vi "AndorTester.vi"() -> ()   [LabVIEW 2014]
uses:
  <userlib>/atmcd32d/Error Code Enum typedef.ctl
  <userlib>/atmcd32d/ReadMode_mode typedef.ctl
  <userlib>/atmcd32d/AcquisitionMode_mode typedef.ctl
panel:
  in  "set temp":i32
  out "status":T1
  out "temperature":i32
  out "Numeric":i32
  out "size(s)":i32
  out "Waveform Chart":i32[](graph)
  in  "stop":bool
  out "Current camera":i32
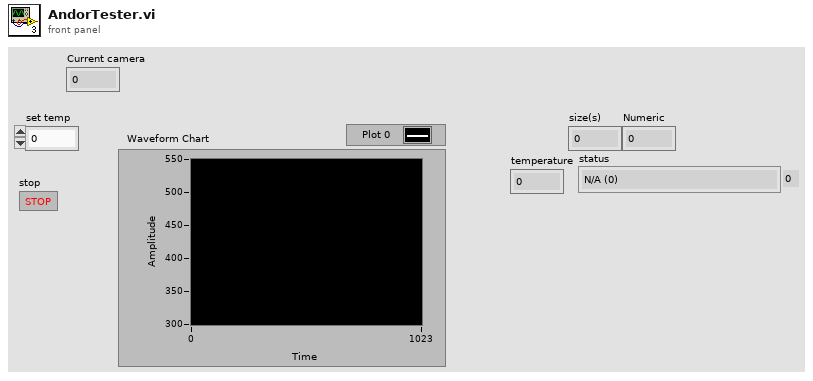
[diagram p1: front panel]
types:
  T1 = typedef "Error Code Enum typedef.ctl" = enum32{"N/A (0)", "DRV_ERROR_CODES", "DRV_SUCCESS", "DRV_VXDNOTINSTALLED", "DRV_ERROR_SCAN", "DRV_ERROR_CHECK_SUM", "DRV_ERROR_FILELOAD", "DRV_UNKNOWN_FUNC", "DRV_ERROR_VXD_INIT", "DRV_ERROR_ADDRESS", "DRV_ERROR_PAGELOCK", "DRV_ERROR_PAGEUNLOCK", "DRV_ERROR_BOARDTEST", "DRV_ERROR_ACK", "DRV_ERROR_UP_FIFO", "DRV_ERROR_PATTERN", "N/A (16)", "DRV_ACQUISITION_ERRORS", "DRV_ACQ_BUFFER", "DRV_ACQ_DOWNFIFO_FULL", "DRV_PROC_UNKONWN_INSTRUCTION", "DRV_ILLEGAL_OP_CODE", "DRV_KINETIC_TIME_NOT_MET", "DRV_ACCUM_TIME_NOT_MET", "DRV_NO_NEW_DATA", "N/A (25)", "DRV_SPOOLERROR", "N/A (27)", "N/A (28)", "N/A (29)", "N/A (30)", "N/A (31)", "N/A (32)", "DRV_TEMPERATURE_CODES", "DRV_TEMPERATURE_OFF", "DRV_TEMPERATURE_NOT_STABILIZED", "DRV_TEMPERATURE_STABILIZED", "DRV_TEMPERATURE_NOT_REACHED", "DRV_TEMPERATURE_OUT_RANGE", "DRV_TEMPERATURE_NOT_SUPPORTED", "DRV_TEMPERATURE_DRIFT", "N/A (41)", "N/A (42)", "N/A (43)", "N/A (44)", "N/A (45)", "N/A (46)", "N/A (47)", "N/A (48)", "DRV_GENERAL_ERRORS", "DRV_INVALID_AUX", "DRV_COF_NOTLOADED", "DRV_FPGAPROG", "DRV_FLEXERROR", "DRV_GPIBERROR", "N/A (55)", "N/A (56)", "N/A (57)", "N/A (58)", "N/A (59)", "N/A (60)", "N/A (61)", "N/A (62)", "N/A (63)", "DRV_DATATYPE", "DRV_DRIVER_ERRORS", "DRV_P1INVALID", "DRV_P2INVALID", "DRV_P3INVALID", "DRV_P4INVALID", "DRV_INIERROR", "DRV_COFERROR", "DRV_ACQUIRING", "DRV_IDLE", "DRV_TEMPCYCLE", "DRV_NOT_INITIALIZED", "DRV_P5INVALID", "DRV_P6INVALID", "DRV_INVALID_MODE", "DRV_INVALID_FILTER", "DRV_I2CERRORS", "DRV_I2CDEVNOTFOUND", "DRV_I2CTIMEOUT", "DRV_P7INVALID", "N/A (84)", "N/A (85)", "N/A (86)", "N/A (87)", "N/A (88)", "N/A (89)", "DRV_IOCERROR", "DRV_VRMVERSIONERROR"}
  T2 = typedef "AcquisitionMode_mode typedef.ctl" = enum16{"Reserved (0)", "Single Scan", "Accumulate", "Kinetics", "Fast Kinetics", "Run Till Abort", "Reserved (6)", "Reserved (7)", "Reserved (8)", "Time Delayed Integration"}
  T3 = typedef "ReadMode_mode typedef.ctl" = enum16{"Full Vertical Binning", "Multi-Track", "Random-Track", "Single-Track", "Image"}
  T4 = typedef "IMAQ Image.ctl" = refnum<image>
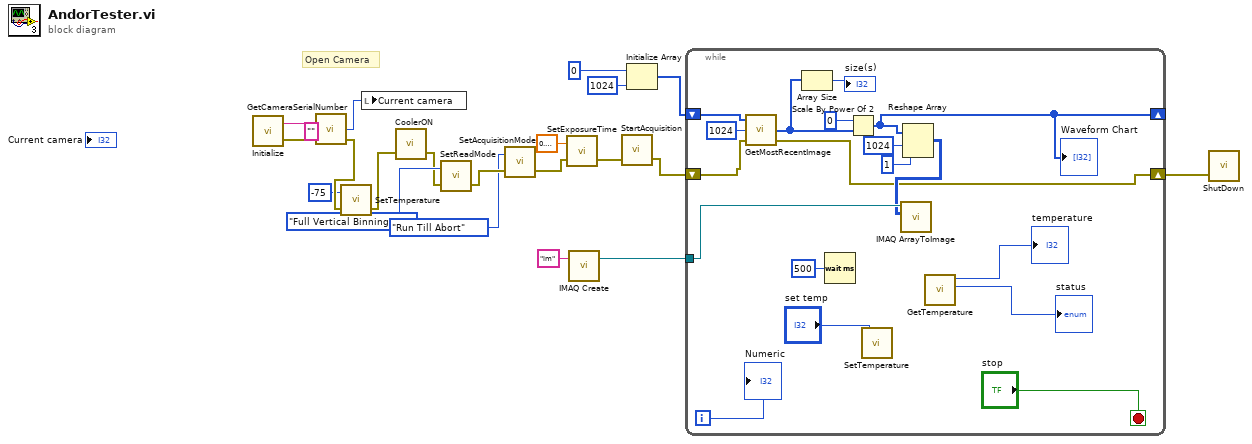
[diagram p0: block diagram]
diagram:
  # "Open Camera"
  n1 = call <userlib>:"Initialize.vi"("directory (\"\")"="" ("directory (\"\")")) -> ("error out"=w18:errorcluster)  [unwired: 1 in, 1 out]
  n2 = call <userlib>:"GetCameraSerialNumber.vi"("error in (no error)"=w18) -> ("error out"=w3:errorcluster, "number"=w19:i32)  [unwired: 2 in, 1 out]
  n3 = call <userlib>:"SetTemperature.vi"("error in (no error)"=w3, "temperature"=-75) -> ("error out"=w2:errorcluster)  [unwired: 1 out]
  n4 = local write "Current camera"(w19) -> ()
  n5 = call <userlib>:"CoolerON.vi"("error in (no error)"=w2) -> ("error out"=w4:errorcluster)  [unwired: 1 in, 1 out]
  n6 = call <userlib>:"SetReadMode.vi"("error in (no error)"=w4, "mode"=ReadMode_mode_typedef."Full Vertical Binning") -> ("error out"=w10:errorcluster)  [unwired: 1 out]
  n7 = call <userlib>:"SetAcquisitionMode.vi"("error in (no error)"=w10, "mode"=AcquisitionMode_mode_typedef."Run Till Abort") -> ("error out"=w7:errorcluster)  [unwired: 1 out]
  n8 = call <userlib>:"SetExposureTime.vi"("error in (no error)"=w7, "time"=sgl 0.3) -> ("error out"=w6:errorcluster)  [unwired: 1 out]
  n9 = call "IMAQ Create"("Image Name"="im") -> ("New Image"=w17:T4)  [unwired: 4 in, 1 out]
  n10 = call <userlib>:"StartAcquisition.vi"("error in (no error)"=w6) -> ("error out"=w5:errorcluster)  [unwired: 1 in, 1 out]
  n11 = Initialize Array(0, 1024 ("dimension size")) -> (w13:i32[])
  n12 = while {
    tunnel: w17 -> [w37]
    shift-right: [w28] -> _
    shift-left: w13 -> [w35]
    shift-right: [w29] -> w11
    shift-left: w5 -> [w30]
    i -> [w24]
    stop <- "stop" stop-if-true
    n13 = call <userlib>:"GetMostRecentImage.vi"("error in (no error)"=w30, "size"=1024, "array"=w35) -> ("error out"=w29:errorcluster, "array"=w27:i32[])  [unwired: 1 out]
    n14 = Array Size(array=w27) -> (size(s)=→"size(s)":i32)
    n15 = Wait (ms)(milliseconds to wait=u32 500) -> ()  [unwired: 1 out]
    n16 = Scale By Power Of 2(n=i16 0, x=w27) -> (x*2^n=w28:i32[])
    "Waveform Chart" <- w28
    n17 = call <userlib>:"SetTemperature.vi"("temperature"="set temp") -> ()  [unwired: 1 in, 2 out]
    n18 = Reshape Array(w28, 1024 ("dimension size"), 1 ("dimension size")) -> (w31:i32[][])
    n19 = call "IMAQ ArrayToImage"("Image Pixels (U8)"=w31, "Image"=w37) -> ()  [unwired: 8 in, 2 out]
    n20 = call <userlib>:"GetTemperature.vi"() -> ("status"=→"status":T1, "temperature"=→"temperature":i32)  [unwired: 4 in, 2 out]
    "Numeric" <- w24
  }
  n21 = call <userlib>:"ShutDown.vi"("error in (no error)"=w11) -> ()  [unwired: 1 in, 2 out]
